vi "Vision_Processing_R_R7.vi"(0 "Current State":T1(ring)=enum."Sub - 4", 1 "Image Dst":T6=refnum, 2 "Inpute Image":T6=refnum, 3 "Startup Flag":bool, 5 "Current ROI Descriptor":T11={"Global Rectangle"=[0, 89, 320, 195], "Contours"=[{"ID"=enum."External", "Type"=12, "Coordinates"=[0, 89, 320, 195, 0]}]} {"Contours"."Type" items=["No Selection", "Point", "Line", "Rectangle", "Oval", "Polygon", "Freehand Region", "Annulus", "Unused2", "Unused3", "Broken Line", "Freehand Line", "Rotated Rectangle"]}, 6 "Avg Score - Last":dbl=887.1599975585938, 7 "error in (no error)":errorcluster, 8 "Current Settings":T9={"Curve Parameters"={"Extraction Mode"=1, "Edge Threshold"=150, "Edge Filter Size"=0, "Min Length"=25, "Row Search Step Size"=15, "Col Search Step Size"=15, "Max Endpoint Gap"=2, "Closed"=TRUE, "Subpixel"=TRUE}, "Match Mode"={"Rotation"=TRUE, "Scale"=TRUE, "Occlusion"=TRUE, "Reserved"=FALSE, "Reserved"=FALSE, "Reserved"=FALSE}, "Range Settings"=[{"Match Constraints"=0, "Min"=-5.0, "Max"=5.0}, {"Match Constraints"=1, "Min"=72.07644500732422, "Max"=86.07644500732422}, {"Match Constraints"=2, "Min"=0.0, "Max"=25.0}], "Number of Matches"=1, "Minimum Match Score"=762.16, "SubPixel Accuracy"=TRUE, "Adv. Geometric Match Options 2"=[{"Setup Data Item"=20, "Item Value"=0.0}, {"Setup Data Item"=22, "Item Value"=1.0}]} {"Curve Parameters"."Extraction Mode" items=["Normal", "Uniform Regions"]; "Curve Parameters"."Edge Filter Size" items=["Fine", "Normal", "Contour Tracing"]; "Curve Parameters"."Max Endpoint Gap" min=0; "Curve Parameters"."Col Search Step Size" min=1 max=255 step=1; "Curve Parameters"."Row Search Step Size" min=1 max=255 step=1; "Curve Parameters"."Min Length" min=0; "Curve Parameters"."Edge Threshold" min=1 max=350 step=1; "Range Settings"."Max" format="%.2f"; "Range Settings"."Min" format="%.2f"; "Range Settings"."Match Constraints" items=["Rotation Angle (degrees)", "Scale Factor (%)", "Occlusion (%)"]; "Adv. Geometric Match Options 2"."Setup Data Item" items=["Curve Extraction Mode", "Curve Edge Threshold", "Curve Edge Filter Size", "Min Curve Length", "Curve Row Search Step Size", "Curve Col Search Step Size", "Curve Max Endpoint Gap", "Extract Closed Curves", "Enable Subpixel Curve Extraction", "Enable Correlation Score", "Enable Subpixel Accuracy", "Subpixel Iterations", "Subpixel Tolerance", "Initial Match List Length", "Enable Target Template Curve Score", "Min Match Separation Distance", "Min Match Separation Angle", "Min Match Separation Scale", "Max Match Overlap", "Enable Coarse Result", "Enable Calibration Support", "Enable Contrast Reversal", "Search Strategy", "Refinement Match Factor", "Subpixel Match Factor"]}, 9 "Sub Beacon Search Enable":bool[](array[boolean])=[FALSE, FALSE, FALSE, FALSE, FALSE], 10 "History Data - IN":T5={"Valid Beacon History - in"=[TRUE, TRUE, FALSE, FALSE, FALSE, TRUE, TRUE, TRUE, TRUE, TRUE, TRUE, TRUE, FALSE, FALSE, FALSE, FALSE, TRUE, FALSE, FALSE, FALSE], "Valid Score History"=[879.34375, 873.4494018554688, 0.0, 0.0, 0.0, 885.4176635742188, 901.1104125976562, 896.478759765625, 963.698974609375, 961.74267578125, 933.7388305664062, 839.6618041992188, 0.0, 0.0, 0.0, 0.0, 859.6193237304688, 0.0, 0.0, 0.0], "Valid Scale History"=[79.11884307861328, 79.14892578125, 0.0, 0.0, 0.0, 79.17522430419922, 78.96813201904297, 78.97109985351562, 79.82025909423828, 79.97138214111328, 81.67668151855469, 87.35909271240234, 0.0, 0.0, 0.0, 0.0, 84.73904418945312, 0.0, 0.0, 0.0]} {"Valid Scale History" format="%#_13g"; "Valid Score History" format="%#_13g"}, 13 "Avg Scale - Last":dbl=79.07644500732422, 16 "History Size":i32=20) -> (11 "Avg Scale":dbl=79.07644500732422, 12 "Avg Score":dbl=887.1599975585938, 14 "Tracking Info":T2={"Tracking Coordinates"={"X"=156.85031127929688, "Y"=142.00376892089844}, "Current Valid"=TRUE, "Current State - Out"=enum."Sub - 4"}, 15 "Next Main ROI Descriptor":T3={"Global Rectangle"=[0, 89, 320, 195], "Contours"=[{"ID"=enum."External", "Type"=12, "Coordinates"=[0, 89, 320, 195, 0]}]} {"Contours"."Type" items=["No Selection", "Point", "Line", "Rectangle", "Oval", "Polygon", "Freehand Region", "Annulus", "Unused2", "Unused3", "Broken Line", "Freehand Line", "Rotated Rectangle"]}, 17 "Beacon - Scales":sgl[](array[numeric])=[0.0, 73.4989, 77.23492, 78.247925, 80.65565], 18 "History Data - Out":T4={"Valid Beacon History\nOut"=[TRUE, TRUE, FALSE, FALSE, FALSE, TRUE, TRUE, TRUE, TRUE, TRUE, TRUE, TRUE, FALSE, FALSE, FALSE, FALSE, TRUE, FALSE, FALSE, FALSE], "Valid Score History\nOut"=[879.34375, 873.4494018554688, 0.0, 0.0, 0.0, 885.4176635742188, 901.1104125976562, 896.478759765625, 963.698974609375, 961.74267578125, 933.7388305664062, 839.6618041992188, 0.0, 0.0, 0.0, 0.0, 859.6193237304688, 0.0, 0.0, 0.0], "Valid Scale History\nOut"=[79.11884307861328, 79.14892578125, 0.0, 0.0, 0.0, 79.17522430419922, 78.96813201904297, 78.97109985351562, 79.82025909423828, 79.97138214111328, 81.67668151855469, 87.35909271240234, 0.0, 0.0, 0.0, 0.0, 84.73904418945312, 0.0, 0.0, 0.0]} {"Valid Scale History\nOut" format="%#_13g"; "Valid Score History\nOut" format="%#_13g"}, 19 "Y Coordinates":sgl[](array[numeric])=[0.0, 140.53621, 143.21667, 142.6294, 143.7858], 20 "Beacons Found":bool[](array[boolean])=[FALSE, TRUE, TRUE, TRUE, TRUE], 21 "X Coordinates":sgl[](array[numeric])=[0.0, 80.34589, 131.11809, 182.08443, 236.72212], 22 "Next State":T1(ring)=enum."Sub - 4", 23 "Lock Status":bool=TRUE, 24 "Startup Flag - out":bool, 25 "New Settings":T9={"Curve Parameters"={"Extraction Mode"=1, "Edge Threshold"=150, "Edge Filter Size"=0, "Min Length"=25, "Row Search Step Size"=15, "Col Search Step Size"=15, "Max Endpoint Gap"=2, "Closed"=TRUE, "Subpixel"=TRUE}, "Match Mode"={"Rotation"=TRUE, "Scale"=TRUE, "Occlusion"=TRUE, "Reserved"=FALSE, "Reserved"=FALSE, "Reserved"=FALSE}, "Range Settings"=[{"Match Constraints"=0, "Min"=-5.0, "Max"=5.0}, {"Match Constraints"=1, "Min"=72.07644500732422, "Max"=86.07644500732422}, {"Match Constraints"=2, "Min"=0.0, "Max"=25.0}], "Number of Matches"=1, "Minimum Match Score"=762.16, "SubPixel Accuracy"=TRUE, "Adv. Geometric Match Options 2"=[{"Setup Data Item"=20, "Item Value"=0.0}, {"Setup Data Item"=22, "Item Value"=1.0}]} {"Curve Parameters"."Extraction Mode" items=["Normal", "Uniform Regions"]; "Curve Parameters"."Edge Filter Size" items=["Fine", "Normal", "Contour Tracing"]; "Curve Parameters"."Max Endpoint Gap" min=0; "Curve Parameters"."Col Search Step Size" min=1 max=255 step=1; "Curve Parameters"."Row Search Step Size" min=1 max=255 step=1; "Curve Parameters"."Min Length" min=0; "Curve Parameters"."Edge Threshold" min=1 max=350 step=1; "Range Settings"."Max" format="%.2f"; "Range Settings"."Min" format="%.2f"; "Range Settings"."Match Constraints" items=["Rotation Angle (degrees)", "Scale Factor (%)", "Occlusion (%)"]}, 27 "Right Image 2":T6(plugin-control))   [LabVIEW 2015]
uses:
  <vilib>/vision/Image Controls.llb/IMAQ Image.ctl
  <vilib>/vision/Pattern Matching.llb/IMAQ Curve Parameters.ctl
  <vilib>/vision/Pattern Matching.llb/IMAQ Match Range Setting.ctl
panel:
  in  "Sub - 4 - FIle Path":path=path "/home/lvuser/natinst/bin/BeaconTemplates/4_beacons_right.png"
  in  "3 / 2\nTransition Scale":sgl=100.0
  in  "Score\nCushion- tight":dbl=75.0
  in  "Main ROI Decay\nper Fail (Vertical)":i32=5
  in  "ROI_factor(Horiztonal) (2 b)":sgl=2.0
  in  "ROI_factor(vertical) (2 b)":sgl=1.1
  in  "Sub - 2 File Path":path=path "/home/lvuser/natinst/bin/BeaconTemplates/2_beacons_right.png"
  in  "Scale Decay \nFactor":dbl=0.5
  in  "Scale Decay \nFactor":dbl=5.0
  in  "Valid Treshold\nfor Lock":i16=3
  in  "Horiztonall Beacon \nCushion (pixels)":sgl=17.0
  out "New Min Score":dbl=762.1599975585938
  out "New Low Scale":dbl=72.07644500732422
  out "New high Scale":dbl=86.07644500732422
  in  "Absolute\nMinimum Score":dbl=750.0
  in  "Absolute\nMaximum Scale":dbl=300.0
  in  "Absolute\nMinimum Scale":dbl=10.0
  in  "Default No Lock\nSetting Values":T10={"Min Scale"=20.0, "Max Scale"=170.0, "Min Score"=800.0}
  in  "Score\nCushion":dbl=75.0
  in  "Scale \nCushion":dbl=7.0
  in  "5 / 4\nTransition Scale":sgl=78.0
  in  "4 / 3\nTransition Scale":sgl=85.0
  in  "Timeout \nThrehsold":i32=1000
  in  "Main ROI Decay\nper Fail (Horiztonal)":i32=25
  in  "ROI_factor(Horiztonal) (4 & 5 b)":sgl=5.0
  in  "ROI_factor(vertical) (4 & 5 b)":sgl=1.5
  in  "ROI_factor(vertical) (3 b)":sgl=2.7
  in  "ROI_factor(Horiztonal) (3 b)":sgl=2.5
  out "Current  Score":sgl=884.7116
  out "Current  Scale":sgl=79.58931
  in  "Fail Count - In":i32
  in  "Sub Beacon Template File Path - ARRAY":path[](array[path])=[path "/home/lvuser/natinst/bin/BeaconTemplates/Sub1.png", path "/home/lvuser/natinst/bin/BeaconTemplates/Sub2.png", path "/home/lvuser/natinst/bin/BeaconTemplates/Sub3.png", path "/home/lvuser/natinst/bin/BeaconTemplates/Sub4.png", path "/home/lvuser/natinst/bin/BeaconTemplates/Sub5.png"]
  in  "Sub - 3 - FIle Path":path=path "/home/lvuser/natinst/bin/BeaconTemplates/3_beacons_right.png"
  in  "Normal - 5 - File Path":path=path "/home/lvuser/natinst/bin/BeaconTemplates/5_beacons.png"
  # "INPUTS"
  # "FILE PATHS"
  # "CONFIG"
  # "OUTPUTS"
  # "************"
  # "Range"
  # "Range"
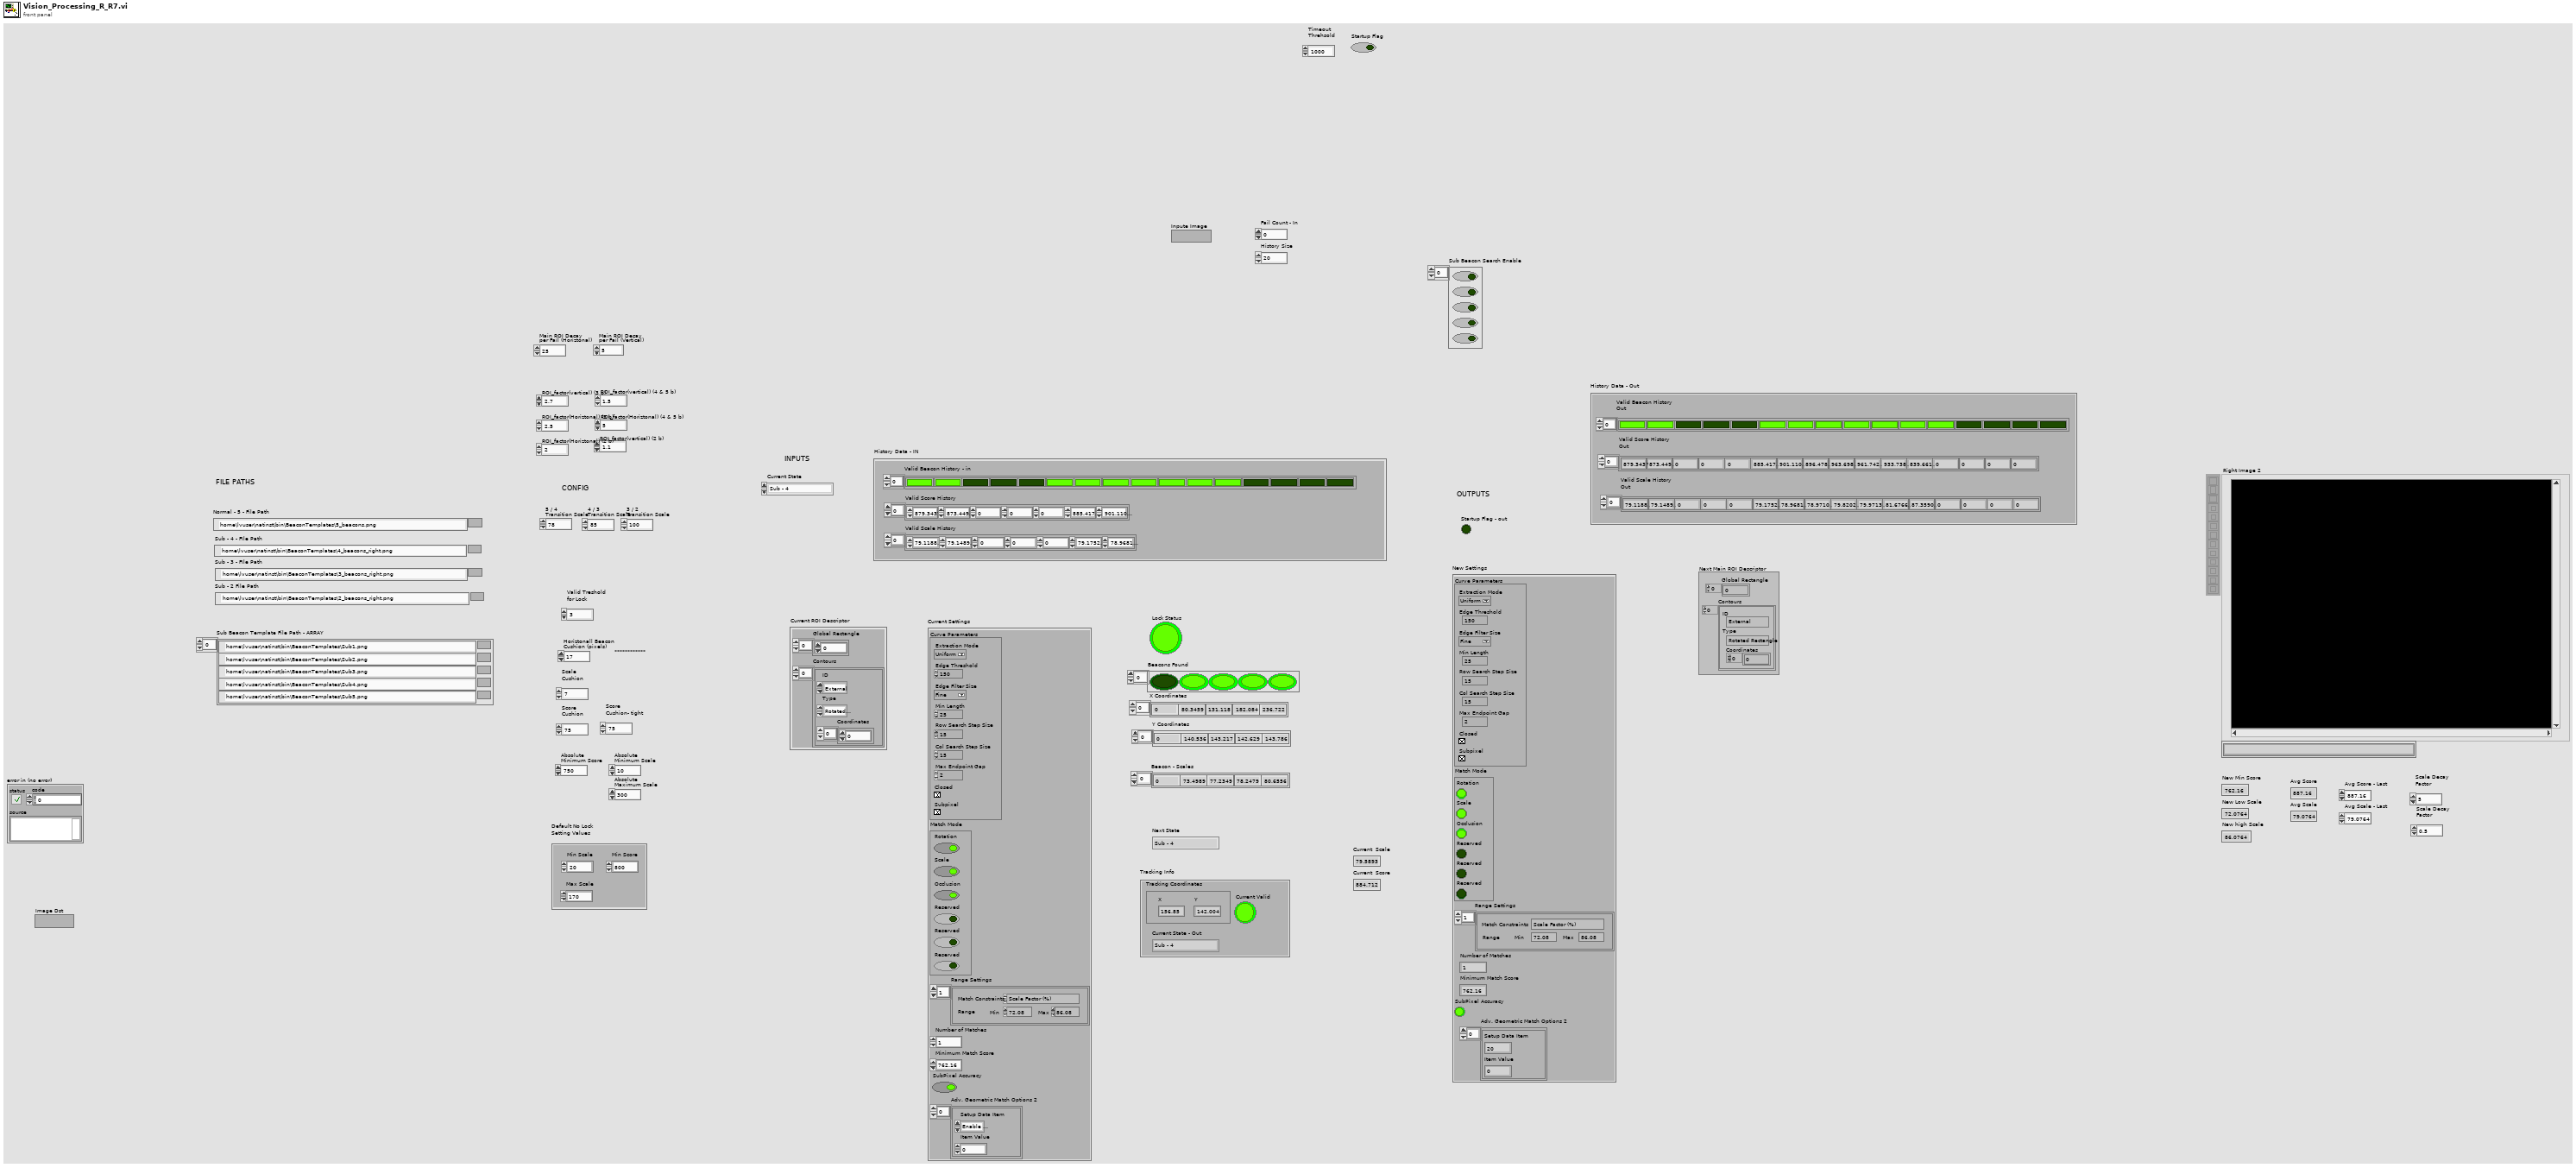
[diagram p1: front panel]
types:
  T1 = enum16{"Sub - 2", "Sub - 3", "Sub - 4", "Normal - 5"}
  T2 = cluster{"Tracking Coordinates":cluster{"X":dbl, "Y":dbl}, "Current Valid":bool, "Current State - Out":enum16{"Sub - 2", "Sub - 3", "Sub - 4", "Normal - 5"}}
  T3 = typedef "ROI Descriptor" = cluster{"Global Rectangle":i32[], "Contours":cluster{"ID":enum32{"External", "Internal"}, "Type":u32, "Coordinates":i32[]}[]}
  T4 = cluster{"Valid Beacon History\nOut":bool[], "Valid Score History\nOut":dbl[], "Valid Scale History\nOut":dbl[]}
  T5 = cluster{"Valid Beacon History - in":bool[], "Valid Score History":dbl[], "Valid Scale History":dbl[]}
  T6 = typedef "IMAQ Image.ctl" = refnum<image>
  T7 = typedef "IMAQ Curve Parameters.ctl" = cluster{"Extraction Mode":u32, "Edge Threshold":i32, "Edge Filter Size":u32, "Min Length":i32, "Row Search Step Size":i32, "Col Search Step Size":i32, "Max Endpoint Gap":i32, "Closed":bool, "Subpixel":bool}
  T8 = typedef "IMAQ Match Range Setting.ctl" = cluster{"Match Constraints":u32, "Min":dbl, "Max":dbl}
  T9 = cluster{"Curve Parameters":T7, "Match Mode":cluster{"Rotation":bool, "Scale":bool, "Occlusion":bool, "Reserved":bool, "Reserved":bool, "Reserved":bool}, "Range Settings":T8[], "Number of Matches":i32, "Minimum Match Score":sgl, "SubPixel Accuracy":bool, "Adv. Geometric Match Options 2":cluster{"Setup Data Item":u16, "Item Value":dbl}[]}
  T10 = cluster{"Min Scale":dbl, "Max Scale":dbl, "Min Score":dbl}
  T11 = cluster{"Global Rectangle":i32[], "Contours":cluster{"ID":enum32{"External", "Internal"}, "Type":u32, "Coordinates":i32[]}[]}
  T12 = typedef "IMAQ GM Match Report.ctl" = cluster{"Position":cluster{"x":sgl, "y":sgl}, "Angle":sgl, "Scale":sgl, "Score":sgl, "Bounding Box":cluster{"x":sgl, "y":sgl}[], "Contrast Reversed":bool, "Occlusion %":sgl, "Template Target Curve Score":sgl, "Target Template Curve Score":sgl, "Correlation Score":sgl}
  T13 = cluster{"Matches (Geometric Matching 1)[0]":T12, "Matches (Geometric Matching 1)[1]":T12, "Matches (Geometric Matching 1)[2]":T12, "Matches (Geometric Matching 1)[3]":T12, "Matches (Geometric Matching 1)[4]":T12, "Matches (Geometric Matching 1)[5]":T12, "Matches (Geometric Matching 1)[6]":T12, "Matches (Geometric Matching 1)[7]":T12, "Matches (Geometric Matching 1)[8]":T12}
  T14 = cluster{"Bounding Box[0]":cluster{"x":sgl, "y":sgl}, "Bounding Box[1]":cluster{"x":sgl, "y":sgl}, "Bounding Box[2]":cluster{"x":sgl, "y":sgl}, "Bounding Box[3]":cluster{"x":sgl, "y":sgl}, "Bounding Box[4]":cluster{"x":sgl, "y":sgl}, "Bounding Box[5]":cluster{"x":sgl, "y":sgl}, "Bounding Box[6]":cluster{"x":sgl, "y":sgl}, "Bounding Box[7]":cluster{"x":sgl, "y":sgl}, "Bounding Box[8]":cluster{"x":sgl, "y":sgl}}
  T15 = cluster{"Position":cluster{"x":sgl, "y":sgl}, bool, "Current State - Out":enum16{"Sub - 2", "Sub - 3", "Sub - 4", "Normal - 5"}}
  T16 = cluster{"Position":cluster{"x":sgl, "y":sgl}, bool, "Current State":enum16{"Sub - 2", "Sub - 3", "Sub - 4", "Normal - 5"}}
  T17 = typedef "IMAQ Rectangle" = cluster{"Left":i32, "Top":i32, "Right":i32, "Bottom":i32, "Rotation":dbl}
  T18 = cluster{"index":u32, "Min Scale":dbl, "Max Scale":dbl}
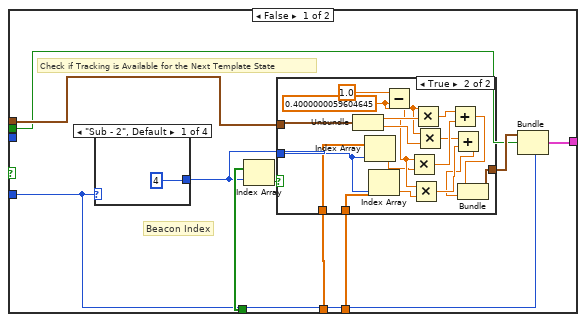
[diagram p2: hidden frame]
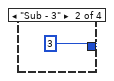
[diagram p4: hidden frame]
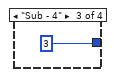
[diagram p5: hidden frame]
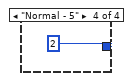
[diagram p6: hidden frame]
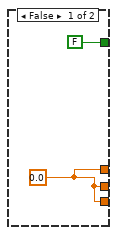
[diagram p7: hidden frame]
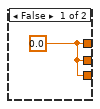
[diagram p8: hidden frame]
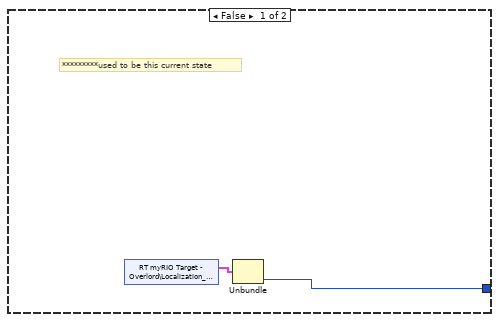
[diagram p12: hidden frame]
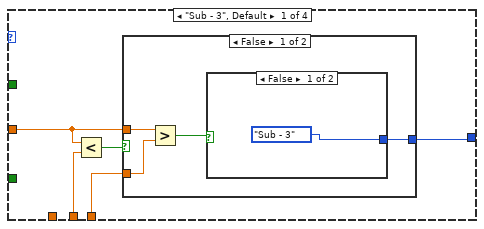
[diagram p13: hidden frame]
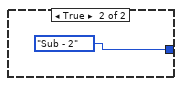
[diagram p14: hidden frame]
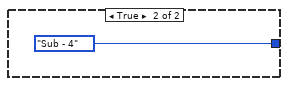
[diagram p15: hidden frame]
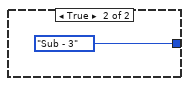
[diagram p16: hidden frame]
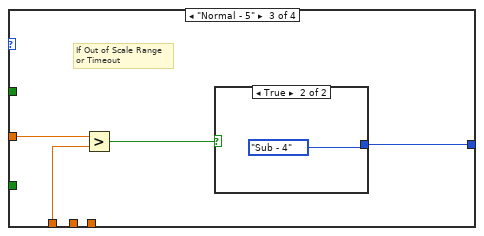
[diagram p17: hidden frame]
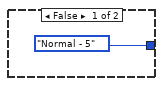
[diagram p18: hidden frame]
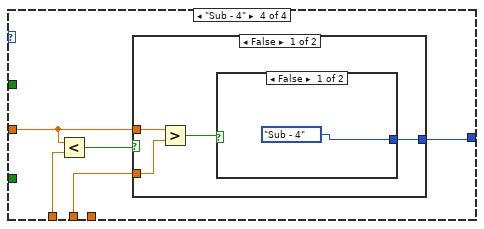
[diagram p19: hidden frame]
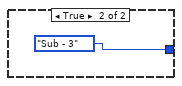
[diagram p20: hidden frame]
diagram:
  (unwired) enum16{"Short Range", "Long Range"}."Short Range"
  # "Next Settings"
  n1 = flat-sequence {
    tunnel: [w8] -> w3
    tunnel: [w7] -> w2
    tunnel: ["Image Dst"] -> w1
    tunnel: w3 -> [w133]
    tunnel: w2 -> [w131]
    tunnel: w1 -> [w132]
    frame #0 {
      # "APPLY FILTERING"
      n2 = call "Camera - Filtering"("Image In"="Inpute Image", "Image Dst"="Image Dst", "error in"="error in (no error)") -> ("Image Out"=w8:T6, "error out"=w7:errorcluster)  [unwired: 23 in]
    }
    frame #1 {
      w95 = u32 1 ("index")
      w116 = u8 5
      # "Start up Template"
      # "Image Lock"
      # "Update Tracking Coordinates"
      # "CURRENT VALID"
      # "*************"
      # "Beacon - Y"
      # "Beacon - X"
      # "Beacons Found"
      # "Build ROI for Individual Beacons Based on Main Bounding Box"
      # "Starting X Lower Bound"
      # "Length of\nIndividual Beacon ROI"
      # "Length of Bounding Box"
      # "Choose ROI Factor based on Next State"
      # "Current Match"
      # "Current ROI"
      # "Image Lock"
      # "Force SR on Startup"
      # "Valid History"
      # "Draw ROI and stuff on outputi mage"
      # "Pull Down Startup IF Already True and Lock\nOtherwise don't update"
      # "Next Settings"
      # "Apply Limits to Settings"
      # "Scale"
      # "Min Score"
      # "Lower Scale"
      # "Upper Scale"
      # "Current Settings"
      # "Current Min\n& Max Scale"
      # "Current Valid"
      # "Update Search Settings"
      # "Update Template State"
      # "Calculate Average Scale/Score"
      # "max avg"
      # "Min Required to use avarage"
      # "Valid  Ccount\n(up to 3)"
      # "****# of previous in history that must be true\nin order for position to be considered \"locked\""
      # "Update Shift Arrays"
      # "# of Beacons Found to be valid"
      # "# of beacons"
      # "Matches"
      # "image out"
      n3 = Select(t=T1."Sub - 2", s="Startup Flag", f="Current State") -> (s? t:f=w18:T1)
      n4 = case shown="\"Sub - 4\"" w18 {
        tunnel: w133 -> [w468 w500 w531 w566]
        tunnel: w132 -> [w467 w499 w530 w565]
        tunnel: "Current ROI Descriptor" -> [w466 w498 w528 w564]
        tunnel: "Current Settings" -> [w465 w497 w527 w563]
        tunnel: [w461 w493 w524 w559] -> w54
        tunnel: [w460 w492 w525 w558] -> w75
        tunnel: [w458 w490 w526 w556] -> w124
        tunnel: w131 -> [_ _ w529 w555]
        tunnel: "Sub Beacon Search Enable" -> [w459 w491 w532 w554]
        tunnel: [sgl 3.0 ("y") sgl 2.0 ("y") 4.0 sgl 5.0 ("y")] -> w129
        tunnel: [w456 w488 w522 w552] -> w128
        tunnel: [2 2 3 4] -> w125
        frame "Sub - 3" {
          n5 = call "Short Range 2"("Image In"=w468, "Image Dst"=w467, "ROI Descriptor (Geometric Matching 1)"=w466, "Settings (Geometric Matching 1)"=w465, "Template File Path (Geometric Matching 1)"="Sub - 3 - FIle Path") -> ("Image Out"=w460:T6, "Matches (Geometric Matching 1)"=w461:T12[], "Number of Matches (Geometric Matching 1)"=w462:i32, "error out"=w456:errorcluster)  [unwired: 19 in]
          n6 = Equal?(x=w462, y=1) -> (x = y?=w463:bool)
          n7 = case shown="True" w463 {
            tunnel: w459 -> [w476 w479]
            tunnel: [w469 w480] -> w458
            frame False {
              w470 = FALSE
              # "F"
              # "No Main Found,\nDon't Search any Subs"
              n8 = Replace Array Subset(array=w476, new element #1=w470, index #1=0 ("y"), new element #2=w470, index #2=1 ("y"), new element #3=w470, index #3=2 ("y"), new element #4=w470, index #4=3 ("y"), new element #5=w470, index #5=4 ("y")) -> (w469:bool[])
            }
            frame True {
              w478 = TRUE
              w477 = FALSE
              n9 = Replace Array Subset(array=w479, new element #1=w477, index #1=0 ("y"), new element #2=w477, index #2=1 ("y"), new element #3=w478, index #3=2 ("y"), new element #4=w478, index #4=3 ("y"), new element #5=w478, index #5=4 ("y")) -> (w480:bool[])
            }
          }
        }
        frame "Sub - 2" {
          n10 = call "Short Range"("Image In"=w500, "Image Dst"=w499, "ROI Descriptor (Geometric Matching 1)"=w498, "Settings (Geometric Matching 1)"=w497, "Template File Path (Geometric Matching 1)"="Sub - 2 File Path") -> ("Image Out"=w492:T6, "Matches (Geometric Matching 1)"=w493:T12[], "Number of Matches (Geometric Matching 1)"=w494:i32, "error out"=w488:errorcluster)  [unwired: 19 in]
          n11 = Equal?(x=w494, y=1) -> (x = y?=w495:bool)
          n12 = case shown="True" w495 {
            tunnel: w491 -> [w508 w511]
            tunnel: [w501 w512] -> w490
            frame False {
              w502 = FALSE
              # "F"
              # "No Main Found,\nDon't Search any Subs"
              n13 = Replace Array Subset(array=w508, new element #1=w502, index #1=0 ("y"), new element #2=w502, index #2=1 ("y"), new element #3=w502, index #3=2 ("y"), new element #4=w502, index #4=3 ("y"), new element #5=w502, index #5=4 ("y")) -> (w501:bool[])
            }
            frame True {
              w510 = TRUE
              w509 = FALSE
              # "Search for specific Beacons"
              n14 = Replace Array Subset(array=w511, new element #1=w509, index #1=0 ("y"), new element #2=w509, index #2=1 ("y"), new element #3=w509, index #3=2 ("y"), new element #4=w510, index #4=3 ("y"), new element #5=w510, index #5=4 ("y")) -> (w512:bool[])
            }
          }
        }
        frame "Sub - 4" {
          # "**Make sure this selects the \nappropriate beacons to search for!!"
          n15 = call "Dumping Range"("Image In"=w531, "Image Dst"=w530, "ROI Descriptor (Geometric Matching 1)"=w528, "Settings (Geometric Matching 1)"=w527, "Template File Path (Geometric Matching 1)"="Sub - 4 - FIle Path", "error in"=w529) -> ("Image Out"=w525:T6, "Matches (Geometric Matching 1)"=w524:T12[], "Number of Matches (Geometric Matching 1)"=w521:i32, "error out"=w522:errorcluster)  [unwired: 18 in]
          n16 = Equal?(x=w521, y=1) -> (x = y?=w519:bool)
          n17 = case shown="True" w519 {
            tunnel: w532 -> [w541 w544]
            tunnel: [w534 w545] -> w526
            frame False {
              w535 = FALSE
              # "F"
              # "No Main Found,\nDon't Search any Subs"
              n18 = Replace Array Subset(array=w541, new element #1=w535, index #1=0 ("y"), new element #2=w535, index #2=1 ("y"), new element #3=w535, index #3=2 ("y"), new element #4=w535, index #4=3 ("y"), new element #5=w535, index #5=4 ("y")) -> (w534:bool[])
            }
            frame True {
              w543 = TRUE
              n19 = Replace Array Subset(array=w544, new element #1=FALSE, index #1=0 ("y"), new element #2=w543, index #2=1 ("y"), new element #3=w543, index #3=2 ("y"), new element #4=w543, index #4=3 ("y"), new element #5=w543, index #5=4 ("y")) -> (w545:bool[])
            }
          }
        }
        frame "Normal - 5" {
          n20 = call "Long Range"("Image In"=w566, "Image Dst"=w565, "ROI Descriptor (Geometric Matching 1)"=w564, "Settings (Geometric Matching 1)"=w563, "Template File Path (Geometric Matching 1)"="Normal - 5 - File Path", "error in"=w555) -> ("Image Out"=w558:T6, "Matches (Geometric Matching 1)"=w559:T12[], "Number of Matches (Geometric Matching 1)"=w561:i32, "error out"=w552:errorcluster)  [unwired: 18 in]
          n21 = Equal?(x=w561, y=1) -> (x = y?=w557:bool)
          n22 = case shown="True" w557 {
            tunnel: w554 -> [w574 w576]
            tunnel: [w567 w575] -> w556
            frame False {
              w568 = FALSE
              # "F"
              # "No Main Found,\nDon't Search any Subs"
              n23 = Replace Array Subset(array=w574, new element #1=w568, index #1=0 ("y"), new element #2=w568, index #2=1 ("y"), new element #3=w568, index #3=2 ("y"), new element #4=w568, index #4=3 ("y"), new element #5=w568, index #5=4 ("y")) -> (w567:bool[])
            }
            frame True {
              w577 = TRUE
              # "T"
              # "Search for ALL Beacons"
              n24 = Replace Array Subset(array=w576, new element #1=w577, index #1=0 ("y"), new element #2=w577, index #2=1 ("y"), new element #3=w577, index #3=2 ("y"), new element #4=w577, index #4=3 ("y"), new element #5=w577, index #5=4 ("y")) -> (w575:bool[])
            }
          }
        }
      }
      n25 = Array To Cluster(array=w54) -> (cluster=w44:T13)
      n26 = Unbundle By Name(w44) -> ("Matches (Geometric Matching 1)[0].Position"=w20:cluster{"x":sgl, "y":sgl}, "Matches (Geometric Matching 1)[0].Bounding Box"=w42:cluster{"x":sgl, "y":sgl}[], "Matches (Geometric Matching 1)[0].Scale"=w74:sgl, "Matches (Geometric Matching 1)[0].Score"=w86:sgl)
      "Current  Scale" <- w74
      "Current  Score" <- w86
      n27 = Array To Cluster(array=w42) -> (cluster=w43:T14)
      n28 = Unbundle By Name(w43) -> ("Bounding Box[0].x"=w33:sgl, "Bounding Box[0].y"=w32:sgl, "Bounding Box[2].x"=w31:sgl, "Bounding Box[2].y"=w30:sgl)
      n29 = Bundle("x"=w33, "y"=w32, "x"=w31, "y"=w30) -> (w28:cluster{"x":sgl, "y":sgl, "x":sgl, "y":sgl})  [unwired: 1 in]
      n30 = call "IMAQ Overlay Rectangle"("Rectangle"=w28, "Image"=w75) -> ("Image Out"=w29:T6)  [unwired: 8 in, 1 out]
      n31 = Subtract(x=w31, y=w33) -> (x-y=w37:sgl)
      n32 = Divide(x=w37, y=w129) -> (x/y=w39:dbl)
      n33 = Multiply(x="Horiztonall Beacon \nCushion (pixels)", y=w74) -> (x*y=w27:sgl)
      n34 = Divide(x=w27, y=sgl 100.0) -> (x/y=w24:sgl)
      n35 = Subtract(x=w32, y=w24) -> (x-y=w40:sgl)
      n36 = Add(x=w24, y=w30) -> (x+y=w41:sgl)
      n37 = for {
        N: 5 -> [_]
        tunnel: w124 -> [w213] mode=indexing
        shift-right: [w207] -> _
        shift-left: w33 -> [w212]
        tunnel: w39 -> [w211]
        tunnel: w40 -> [w204]
        tunnel: w41 -> [w203]
        tunnel: [w210] -> w35 mode=indexing
        tunnel: w24 -> [w205]
        # "Divide Bounding Box"
        # "Upper Bound of Current is\nLower Bound for Next"
        n38 = case shown="True" w213 {
          tunnel: w212 -> [w214 w215]
          tunnel: w211 -> [_ w217]
          tunnel: [w214 w216] -> w207
          tunnel: [w214 w215] -> w209
          frame False {
            # "Don't Care"
          }
          frame True {
            # "X Lower Bound"
            n39 = Add(x=w215, y=w217) -> (x+y=w216:dbl)
          }
        }
        n40 = Subtract(x=w209, y=w205) -> (x-y=w208:dbl)
        n41 = Add(x=w207, y=w205) -> (x+y=w206:dbl)
        n42 = call "Bound_RO_R_R0I.vi"("Bottom Right - Y"=w203, "Right - X"=w206, "Top Left - Y"=w204, "Top  Left - x"=w208) -> ("ROI Descriptor"=w210:T3)  [unwired: 7 in]
      }
      n43 = for {
        N: 5 -> [_]
        tunnel: w75 -> [w182]
        tunnel: w128 -> [w181]
        tunnel: w35 -> [w174] mode=indexing
        tunnel: "Sub Beacon Template File Path - ARRAY" -> [w180] mode=indexing
        tunnel: [w179] -> w12 mode=indexing
        tunnel: [w178] -> w11 mode=indexing
        tunnel: [w177] -> w13 mode=indexing
        tunnel: w124 -> [w176] mode=indexing
        tunnel: "Current Settings" -> [w175]
        shift-right: [w172] -> w76
        shift-left: w29 -> [w173]
        tunnel: [w171] -> w65 mode=indexing
        n44 = case shown="True" w176 {
          tunnel: w182 -> [_ w196]
          tunnel: w181 -> [_ w195]
          tunnel: w174 -> [_ w194]
          tunnel: w180 -> [_ w193]
          tunnel: [w183 w189] -> w179
          tunnel: [w183 w188] -> w178
          tunnel: [FALSE w187] -> w177
          tunnel: w175 -> [_ w186]
          tunnel: [w183 w185] -> w171
          frame False {
            w183 = sgl 0.0 ("x")
          }
          frame True {
            n45 = call "Sub Beacon Pattern Match"("Image In"=w196, "ROI Descriptor (Geometric Matching 1)"=w194, "Settings (Geometric Matching 1)"=w186, "Template File Path (Geometric Matching 1)"=w193, "error in"=w195) -> ("Matches (Geometric Matching 1)"=w190:T12[], "Number of Matches (Geometric Matching 1)"=w191:i32)  [unwired: 19 in, 2 out]
            n46 = Equal?(x=w191, y=1) -> (x = y?=w187:bool)
            n47 = case shown="True" w187 {
              tunnel: w190 -> [_ w201]
              tunnel: [w197 w200] -> w189
              tunnel: [w197 w199] -> w188
              tunnel: [w197 w198] -> w185
              frame False {
                w197 = sgl 0.0 ("x")
              }
              frame True {
                n48 = Array To Cluster(array=w201) -> (cluster=w202:T13)
                n49 = Unbundle By Name(w202) -> ("Matches (Geometric Matching 1)[0].Position.x"=w200:sgl, "Matches (Geometric Matching 1)[0].Position.y"=w199:sgl, "Matches (Geometric Matching 1)[0].Scale"=w198:sgl)
              }
            }
          }
        }
        n50 = call "IMAQ Overlay ROI"("ROI Descriptor"=w174, "Image"=w173) -> ("Image Out"=w172:T6)  [unwired: 8 in, 1 out]
      }
      "Beacons Found" <- w13
      "X Coordinates" <- w12
      "Y Coordinates" <- w11
      "Beacon - Scales" <- w65
      n51 = Boolean To (0,1)(Boolean=w13) -> (0, 1=w126:i16[])
      n52 = Add Array Elements(numeric array=w126) -> (sum=w127:i16)
      n53 = Greater Or Equal?(x=w127, y=w125) -> (x >= y?=w19:bool)
      n54 = case shown="False" w19 {
        tunnel: "Fail Count - In" -> [w452 _]
        tunnel: [w451 u16 0] -> w109
        frame False {
          n55 = Increment(x=w452) -> (x+1=w451:i32)
        }
        frame True {
          # "reset fail count"
        }
      }
      n56 = Unbundle By Name("History Data - IN") -> ("Valid Beacon History - in"=w72:bool[], "Valid Score History"=w71:dbl[], "Valid Scale History"=w70:dbl[])
      n57 = Greater?(x=w109, y="Timeout \nThrehsold") -> (0:w21:bool)
      n58 = Decrement(x="History Size") -> (x-1=w122:i32)
      n59 = for {
        N: "History Size" -> [_]
        shift-right: [w429] -> w69
        shift-left: w72 -> [w417]
        tunnel: w122 -> [w425]
        shift-right: [w422] -> w68
        shift-left: w71 -> [w424]
        shift-right: [w421] -> w67
        shift-left: w70 -> [w423]
        tunnel: w86 -> [w420]
        tunnel: w74 -> [w419]
        tunnel: w19 -> [w418]
        i -> [w428]
        # "Reverse Index"
        n60 = Subtract(x=w425, y=w428) -> (x-y=w426:i32)
        n61 = Equal To 0?(x=w426) -> (x = 0?=w427:bool)
        n62 = case shown="True" w427 {
          tunnel: w426 -> [w430 w449]
          tunnel: w417 -> [w440 w442]
          tunnel: [w438 w441] -> w429
          tunnel: w418 -> [_ w450]
          tunnel: w424 -> [w435 w448]
          tunnel: w423 -> [w434 w447]
          tunnel: [w433 w445] -> w422
          tunnel: [w432 w446] -> w421
          tunnel: w420 -> [_ w444]
          tunnel: w419 -> [_ w443]
          frame False {
            # "Shift Old"
            n63 = Decrement(x=w430) -> (x-1=w431:i32)
            n64 = Index Array(array=w440, index=w431) -> (element=w439:bool)
            n65 = Index Array(array=w435, index=w431) -> (element=w437:dbl)
            n66 = Index Array(array=w434, index=w431) -> (element=w436:dbl)
            n67 = Replace Array Subset(array=w440, new element=w439, index=w430) -> (w438:bool[])
            n68 = Replace Array Subset(array=w435, new element=w437, index=w430) -> (w433:dbl[])
            n69 = Replace Array Subset(array=w434, new element=w436, index=w430) -> (w432:dbl[])
          }
          frame True {
            # "Scale"
            # "Score"
            # "Valid"
            # "insert New"
            n70 = Replace Array Subset(array=w448, new element=w444, index=w449) -> (w445:dbl[])
            n71 = Replace Array Subset(array=w447, new element=w443, index=w449) -> (w446:dbl[])
            n72 = Replace Array Subset(array=w442, new element=w450, index=w449) -> (w441:bool[])
          }
        }
      }
      n73 = Boolean To (0,1)(Boolean=w69) -> (0, 1=w120:i16[])
      n74 = Bundle("Valid Beacon History - in"=w69, "Valid Score History"=w68, "Valid Scale History"=w67) -> (→"History Data - Out":T5)  [unwired: 1 in]
      n75 = Add Array Elements(numeric array=w120) -> (sum=w121:i16)
      n76 = Greater Or Equal?(x=w121, y="Valid Treshold\nfor Lock") -> (x >= y?=w87:bool)
      "Lock Status" <- w87
      n77 = Initialize Array(u8 0, w116) -> (w118:u8[])
      n78 = while {
        shift-right: [w400] -> w114
        shift-left: w118 -> [w402]
        tunnel: w69 -> [w408] mode=indexing
        shift-right: [w406] -> w112
        shift-left: u8 0 -> [w409]
        tunnel: "History Size" -> [w407]
        tunnel: w116 -> [w399]
        i -> [w401]
        stop <- w403 stop-if-true
        # "Grab Last 2 Valid Indexes"
        n79 = case shown="True" w408 {
          tunnel: w409 -> [w411 w413]
          tunnel: [w411 w416] -> w406
          tunnel: w402 -> [w410 w415]
          tunnel: w401 -> [_ w414]
          tunnel: [w410 w412] -> w400
          frame False {
          }
          frame True {
            # "Update Index\nto use"
            # "Increment\nValid Count"
            n80 = Replace Array Subset(array=w415, new element=w414, index=w413) -> (w412:u8[])
            n81 = Increment(x=w413) -> (x+1=w416:u8)
          }
        }
        n82 = Greater?(x=w401, y=w407) -> (0:w404:bool)
        n83 = Greater Or Equal?(x=w406, y=w399) -> (x >= y?=w405:bool)
        n84 = Or(x=w405, y=w404) -> (x .or. y?=w403:bool)
      }
      n85 = Greater?(x=w112, y=u8 2) -> (0:w113:bool)
      n86 = case shown="True" w113 {
        tunnel: w112 -> [_ w383]
        tunnel: w114 -> [_ w389]
        tunnel: w68 -> [_ w388]
        tunnel: w67 -> [_ w387]
        tunnel: ["Avg Score - Last" w381] -> w83
        tunnel: ["Avg Scale - Last" w380] -> w84
        frame False {
        }
        frame True {
          w386 = 0.0
          n87 = for {
            N: w383 -> [_]
            tunnel: w389 -> [w396] mode=indexing
            tunnel: w388 -> [w398]
            tunnel: w387 -> [w397]
            shift-right: [w394] -> w385
            shift-left: w386 -> [w392]
            shift-right: [w395] -> w384
            shift-left: w386 -> [w391]
            # "Fetch Last Valid Values"
            n88 = Index Array(array=w398, index=w396) -> (element=w393:dbl)
            n89 = Index Array(array=w397, index=w396) -> (element=w390:dbl)
            n90 = Add(x=w393, y=w392) -> (x+y=w394:dbl)
            n91 = Add(x=w390, y=w391) -> (x+y=w395:dbl)
          }
          n92 = To Double Precision Float(number=w383) -> (double precision float=w382:dbl)
          n93 = Divide(x=w385, y=w382) -> (x/y=w381:dbl)
          n94 = Divide(x=w384, y=w382) -> (x/y=w380:dbl)
        }
      }
      "Avg Score" <- w83
      "Avg Scale" <- w84
      n95 = case shown="True" w87 {
        tunnel: w21 -> [_ w232]
        tunnel: "4 / 3\nTransition Scale" -> [_ w231]
        tunnel: "5 / 4\nTransition Scale" -> [_ w230]
        tunnel: w84 -> [_ w229]
        tunnel: w87 -> [_ w228]
        tunnel: [w224 w227] -> w9
        tunnel: "3 / 2\nTransition Scale" -> [_ w226]
        frame False {
          # "*********used to be this current state"
          n96 = shared-variable "RT myRIO Target - Overlord\\Localization_Variables_r0.lvlib\\Info - Left"() -> (w225:T2)  [unwired: 1 in, 1 out]
          n97 = Unbundle(w225) -> ("Current State - Out"=w224:T1)  [unwired: 2 out]
        }
        frame True {
          # "Timeout"
          n98 = local read "Current State"() -> (w233:T1)
          n99 = case shown="\"Sub - 2\"" w233 {
            tunnel: w228 -> [_ _ _ _]
            tunnel: w229 -> [w237 w249 w254 w260]
            tunnel: w232 -> [_ _ _ _]
            tunnel: w231 -> [w238 _ _ w259]
            tunnel: w230 -> [_ _ w253 w262]
            tunnel: [w234 w246 w252 w258] -> w227
            tunnel: w226 -> [w235 w248 _ _]
            frame "Sub - 3", Default {
              n100 = Less?(x=w237, y=w238) -> (x < y?=w236:bool)
              n101 = case shown="False" w236 {
                tunnel: w237 -> [w242 _]
                tunnel: [w239 T1."Sub - 4"] -> w234
                tunnel: w235 -> [w241 _]
                frame False {
                  n102 = Greater?(x=w242, y=w241) -> (0:w240:bool)
                  n103 = case shown="False" w240 {
                    tunnel: [T1."Sub - 3" T1."Sub - 2"] -> w239
                    frame False {
                    }
                    frame True {
                    }
                  }
                }
                frame True {
                }
              }
            }
            frame "Sub - 2" {
              n104 = Less?(x=w249, y=w248) -> (x < y?=w247:bool)
              n105 = case shown="False" w247 {
                tunnel: [T1."Sub - 2" T1."Sub - 3"] -> w246
                frame False {
                }
                frame True {
                }
              }
            }
            frame "Normal - 5" {
              # "If Out of Scale Range\nor Timeout"
              n106 = Greater?(x=w254, y=w253) -> (0:w255:bool)
              n107 = case shown="True" w255 {
                tunnel: [T1."Normal - 5" T1."Sub - 4"] -> w252
                frame False {
                }
                frame True {
                }
              }
            }
            frame "Sub - 4" {
              n108 = Less?(x=w260, y=w262) -> (x < y?=w261:bool)
              n109 = case shown="False" w261 {
                tunnel: w260 -> [w266 _]
                tunnel: [w263 T1."Normal - 5"] -> w258
                tunnel: w259 -> [w265 _]
                frame False {
                  n110 = Greater?(x=w266, y=w265) -> (0:w264:bool)
                  n111 = case shown="False" w264 {
                    tunnel: [T1."Sub - 4" T1."Sub - 3"] -> w263
                    frame False {
                    }
                    frame True {
                    }
                  }
                }
                frame True {
                }
              }
            }
          }
        }
      }
      "Next State" <- w9
      n112 = local read "Current State"() -> (w15:T1)
      n113 = Equal?(x=w15, y=w9) -> (x = y?=w10:bool)
      n114 = case shown="True" w10 {
        tunnel: w20 -> [w138 w170]
        tunnel: w19 -> [w135 w169]
        tunnel: w18 -> [_ w168]
        tunnel: [w134 w167] -> w14
        tunnel: w9 -> [w141 _]
        tunnel: w13 -> [w143 _]
        tunnel: w12 -> [w140 _]
        tunnel: w11 -> [w139 _]
        frame False {
          # "Beacon Index"
          # "Check if Tracking is Available for the Next Template State"
          n115 = case shown="\"Sub - 2\", Default" w141 {
            tunnel: [4 3 3 2] -> w137
            frame "Sub - 2", Default {
            }
            frame "Sub - 3" {
            }
            frame "Sub - 4" {
            }
            frame "Normal - 5" {
            }
          }
          n116 = Index Array(array=w143, index=w137) -> (element=w142:bool)
          n117 = case shown="True" w142 {
            tunnel: w140 -> [_ w162]
            tunnel: w139 -> [_ w161]
            tunnel: [w144 w158] -> w136
            tunnel: w138 -> [w144 w159]
            tunnel: w137 -> [_ w160]
            frame False {
            }
            frame True {
              w155 = sgl 0.4 ("y")
              n118 = Unbundle(w159) -> ("x"=w156:sgl, "y"=w154:sgl)
              n119 = Index Array(array=w162, index=w160) -> (element=w151:sgl)
              n120 = Index Array(array=w161, index=w160) -> (element=w152:sgl)
              n121 = Subtract(x=sgl 1.0, y=w155) -> (x-y=w153:sgl)
              n122 = Multiply(x=w153, y=w151) -> (x*y=w149:sgl)
              n123 = Multiply(x=w153, y=w152) -> (x*y=w147:sgl)
              n124 = Multiply(x=w155, y=w156) -> (x*y=w150:sgl)
              n125 = Multiply(x=w155, y=w154) -> (x*y=w148:sgl)
              n126 = Add(x=w150, y=w149) -> (x+y=w146:sgl)
              n127 = Add(x=w148, y=w147) -> (x+y=w145:sgl)
              n128 = Bundle(w146, w145) -> (w158:cluster{sgl, sgl})  [unwired: 1 in]
            }
          }
          n129 = Bundle("Position"=w136, w135, "Current State - Out"=w141) -> (w134:T15)  [unwired: 1 in]
        }
        frame True {
          n130 = Bundle("Position"=w170, w169, "Current State"=w168) -> (w167:T16)  [unwired: 1 in]
        }
      }
      "Tracking Info" <- w14
      n131 = Unbundle By Name("Current Settings") -> ("Minimum Match Score"=w106:sgl, "Range Settings"=w92:T8[])
      n132 = case shown="\"Sub - 3\"" w9 {
        tunnel: "ROI_factor(vertical) (3 b)" -> [_ _ w223]
        tunnel: "ROI_factor(Horiztonal) (3 b)" -> [_ _ w222]
        tunnel: "ROI_factor(vertical) (4 & 5 b)" -> [_ w221 _]
        tunnel: "ROI_factor(Horiztonal) (4 & 5 b)" -> [_ w220 _]
        tunnel: "ROI_factor(vertical) (2 b)" -> [w219 _ _]
        tunnel: "ROI_factor(Horiztonal) (2 b)" -> [w218 _ _]
        tunnel: [w219 w221 w223] -> w47
        tunnel: [w218 w220 w222] -> w46
        frame "Sub - 2" {
        }
        frame "Sub - 4", Default {
        }
        frame "Sub - 3" {
        }
      }
      n133 = Index Array(array=w92, index=u32 1) -> (element=w105:T8)
      n134 = Unbundle(w105) -> ("Min"=w103:dbl, "Max"=w102:dbl)  [unwired: 1 out]
      n135 = case shown="True" w87 {
        tunnel: w19 -> [_ w316]
        tunnel: w83 -> [w283 w315]
        tunnel: w84 -> [w282 w314]
        tunnel: w106 -> [_ w313]
        tunnel: w103 -> [_ w312]
        tunnel: w102 -> [_ w311]
        tunnel: [w281 w302] -> w93
        tunnel: [w280 w301] -> w58
        tunnel: [w279 w300] -> w59
        tunnel: "Scale \nCushion" -> [w285 w310]
        tunnel: "Score\nCushion" -> [w284 w309]
        tunnel: "Scale Decay \nFactor" -> [_ w308]
        tunnel: "Scale Decay \nFactor" -> [_ w307]
        tunnel: "Current ROI Descriptor" -> [_ w303]
        tunnel: w54 -> [_ w304]
        tunnel: w47 -> [_ w306]
        tunnel: w46 -> [_ w305]
        tunnel: [w272 w299] -> w45
        tunnel: w10 -> [_ w294]
        tunnel: w9 -> [_ w293]
        frame False {
          # "Initial ROI Descriptor"
          # "Apply No Lock Default for each Template"
          n136 = Unbundle By Name("Default No Lock\nSetting Values") -> ("Min Score"=w281:dbl, "Min Scale"=w280:dbl, "Max Scale"=w279:dbl)
          n137 = disable-structure shown="Disabled" {
            disable-tunnel: [w292 _] -> _
            disable-tunnel: [w291 _] -> _
            disable-tunnel: w285 -> [w290 _]
            disable-tunnel: w284 -> [w289 _]
            disable-tunnel: w283 -> [w288 _]
            disable-tunnel: w282 -> [w287 _]
            frame Disabled {
              n138 = Subtract(x=w288, y=w289) -> ()  [unwired: 1 out]
              n139 = Subtract(x=w287, y=w290) -> (x-y=w292:dbl)
              n140 = Add(x=w290, y=w287) -> (x+y=w291:dbl)
            }
            frame Enabled {
            }
          }
          n141 = Bundle(0, 0, 640, 480, 0) -> (w278:cluster{i32, i32, i32, i32, i32})  [unwired: 1 in]
          n142 = call "IMAQ Convert Rectangle to ROI"("Rectangle"=w278) -> ("ROI Descriptor"=w272:T3)  [unwired: 8 in, 1 out]
        }
        frame True {
          # "Apply Limits to ROI"
          n143 = case shown="True" w316 {
            tunnel: w315 -> [_ w363]
            tunnel: [w331 w360] -> w302
            tunnel: w314 -> [_ w362]
            tunnel: [w330 w340] -> w301
            tunnel: [w329 w339] -> w300
            tunnel: w312 -> [w336 _]
            tunnel: w311 -> [w335 _]
            tunnel: w313 -> [w334 _]
            tunnel: w310 -> [_ w342]
            tunnel: w309 -> [_ w361]
            tunnel: w308 -> [w333 _]
            tunnel: w307 -> [w332 _]
            tunnel: w306 -> [_ w351]
            tunnel: w305 -> [_ w350]
            tunnel: w304 -> [_ w349]
            tunnel: [w320 w338] -> w298
            tunnel: [w319 w348] -> w297
            tunnel: [w318 w337] -> w296
            tunnel: [w317 w347] -> w295
            tunnel: w303 -> [w327 _]
            tunnel: w294 -> [_ w345]
            tunnel: w293 -> [_ w344]
            frame False {
              # "Decrement Score by"
              n144 = Subtract(x=w336, y=w332) -> (x-y=w330:dbl)
              n145 = Add(x=w332, y=w335) -> (x+y=w329:dbl)
              n146 = Subtract(x=w334, y=w333) -> (x-y=w331:dbl)
              n147 = call "IMAQ Convert ROI to Rectangle"("ROI Descriptor"=w327) -> ("Rectangle"=w328:T17)  [unwired: 8 in, 1 out]
              n148 = Unbundle By Name(w328) -> ("Left"=w324:i32, "Top"=w323:i32, "Right"=w322:i32, "Bottom"=w321:i32)
              n149 = Subtract(x=w324, y="Main ROI Decay\nper Fail (Horiztonal)") -> (x-y=w320:i32)
              n150 = Add(x=w322, y="Main ROI Decay\nper Fail (Horiztonal)") -> (x+y=w318:i32)
              n151 = Add(x=w321, y="Main ROI Decay\nper Fail (Vertical)") -> (x+y=w317:i32)
              n152 = Subtract(x=w323, y="Main ROI Decay\nper Fail (Vertical)") -> (x-y=w319:i32)
            }
            frame True {
              # "if switching states"
              # "Scale / Score"
              # "Main ROI"
              # "Horizontal Scale \n(smaller number = smaller ROI)"
              n153 = Subtract(x=w363, y=w361) -> (x-y=w360:dbl)
              n154 = Subtract(x=w362, y=w342) -> (x-y=w341:dbl)
              n155 = Add(x=w342, y=w362) -> (x+y=w343:dbl)
              n156 = Not(x=w345) -> (.not. x?=w346:bool)
              n157 = Array To Cluster(array=w349) -> (cluster=w359:T13)
              n158 = Unbundle By Name(w359) -> ("Matches (Geometric Matching 1)[0].Position.x"=w353:sgl, "Matches (Geometric Matching 1)[0].Position.y"=w355:sgl, "Matches (Geometric Matching 1)[0].Scale"=w354:sgl)
              n159 = Divide(x=w354, y=w351) -> (x/y=w356:sgl)
              n160 = Multiply(x=w354, y=w350) -> (x*y=w358:sgl)
              n161 = Divide(x=w358, y=sgl 2.0) -> (x/y=w352:sgl)
              n162 = Add(x=w355, y=w356) -> (x+y=w347:sgl)
              n163 = Subtract(x=w355, y=w356) -> (x-y=w348:sgl)
              n164 = Subtract(x=w353, y=w352) -> (x-y=w338:sgl)
              n165 = Add(x=w352, y=w353) -> (x+y=w337:sgl)
              n166 = case shown="True" w346 {
                tunnel: w344 -> [_ _]
                tunnel: [w366 w375] -> w339
                tunnel: w343 -> [w366 w377]
                tunnel: [w367 w374] -> w340
                tunnel: w341 -> [w367 w376]
                tunnel: w342 -> [_ w373]
                tunnel: [w365 w370] -> _
                tunnel: w338 -> [w365 w371]
                tunnel: [w364 w369] -> _
                tunnel: w337 -> [w364 w372]
                frame False {
                }
                frame True {
                  w368 = sgl 50.0 ("y")
                  # "Double scale cushion\nif changing states"
                  n167 = Add(x=w377, y=w373) -> (x+y=w375:dbl)
                  n168 = Subtract(x=w376, y=w373) -> (x-y=w374:dbl)
                  n169 = Subtract(x=w371, y=w368) -> (x-y=w370:sgl)
                  n170 = Add(x=w368, y=w372) -> (x+y=w369:sgl)
                }
              }
            }
          }
          n171 = call "Bound_RO_R_R0I.vi"("Bottom Right - Y"=w295, "Right - X"=w296, "Top Left - Y"=w297, "Top  Left - x"=w298) -> ("ROI Descriptor"=w299:T3)  [unwired: 7 in]
        }
      }
      "Next Main ROI Descriptor" <- w45
      n172 = And(x="Startup Flag", y=w87) -> (x .and. y?=w90:bool)
      n173 = case shown="True" w90 {
        tunnel: "Startup Flag" -> [w270 _]
        tunnel: [w270 FALSE] -> w89
        frame False {
        }
        frame True {
        }
      }
      "Startup Flag - out" <- w89
      n174 = Less?(x=w93, y="Absolute\nMinimum Score") -> (x < y?=w97:bool)
      n175 = Less?(x=w58, y="Absolute\nMinimum Scale") -> (x < y?=w61:bool)
      n176 = Greater?(x=w59, y="Absolute\nMaximum Scale") -> (0:w56:bool)
      n177 = Greater?(x=w58, y=w59) -> (0:w62:bool)
      n178 = Less?(x=w59, y=w58) -> (x < y?=w57:bool)
      n179 = Select(t="Absolute\nMinimum Score", s=w97, f=w93) -> (s? t:f=w99:dbl)
      "New Min Score" <- w99
      n180 = Or(x=w61, y=w62) -> (x .or. y?=w63:bool)
      n181 = Or(x=w56, y=w57) -> (x .or. y?=w60:bool)
      n182 = Select(t="Absolute\nMinimum Scale", s=w63, f=w58) -> (s? t:f=w77:dbl)
      "New Low Scale" <- w77
      n183 = Select(t="Absolute\nMaximum Scale", s=w60, f=w59) -> (s? t:f=w78:dbl)
      "New high Scale" <- w78
      n184 = Bundle("index"=w95, "Min Scale"=w77, "Max Scale"=w78) -> (w94:T18)  [unwired: 1 in]
      n185 = Replace Array Subset(array=w92, new element=w94, index=w95) -> (w96:T8[])
      n186 = call "IMAQ Overlay ROI"("ROI Descriptor"=w45, "Image"=w76) -> ("Image Out"=→"Right Image 2":T6)  [unwired: 8 in, 1 out]
      n187 = Bundle By Name(cluster="Current Settings", "Range Settings"=w96, "Minimum Match Score"=w99) -> (→"New Settings":T9)
    }
  }
